vi "Autonics_GetPos.vi"(8 "error in (no error)":errorcluster, 10 "Travel per Pulse (mm)":dbl=0.002, 11 "VISA resource name":refnum<visa-resource-name>) -> (0 "error out":errorcluster, 2 "Current  Position (mm)":dbl format="%#_4g", 3 "VISA resource name out":refnum<visa-resource-name>)   [LabVIEW 2018]
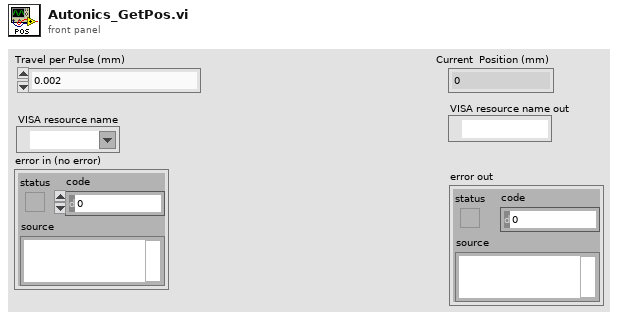
[diagram p1: front panel]
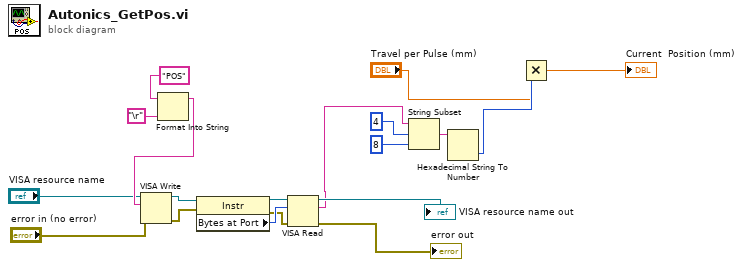
[diagram p0: block diagram]
diagram:
  n1 = Format Into String(initial string="POS" ("string"), "\r") -> (resulting string=w12:string)  [unwired: 2 in, 1 out]
  n2 = VISA Write(VISA resource name="VISA resource name", write buffer=w12, error in (no error)="error in (no error)") -> (VISA resource name out=w16:refnum<visa-resource-name>, error out=w15:errorcluster)  [unwired: 1 out]
  n3 = property class="Instr"(reference=w16, error in=w15) -> (reference out=w19:refnum<visa-resource-name>, error out=w17:errorcluster, "Bytes at Port"=w18:u32)
  n4 = VISA Read(VISA resource name=w19, byte count=w18, error in (no error)=w17) -> (VISA resource name out=→"VISA resource name out":refnum<visa-resource-name>, read buffer=w7:string, error out=→"error out":errorcluster)  [unwired: 1 out]
  n5 = String Subset(string=w7, offset (0)=4, length (rest)=8 ("length (rest)")) -> (substring=w4:string)
  n6 = Hexadecimal String To Number(string=w4) -> (number=w5:u32)  [unwired: 2 in, 1 out]
  n7 = Multiply(x="Travel per Pulse (mm)", y=w5) -> (x*y=→"Current  Position (mm)":dbl)
